vi "_AppData.Test Class.vi"() -> ()   [LabVIEW 2024, in "EQMF.lvlib" / "Config Utils.lvlib"]
uses:
  Config Utils.lvlib
  Class.AppData.lvclass
  <vilib>/Utility/sysdir.llb/System Directory Type.ctl
panel:
  out "App Data Folder":path
  out "Replaced 3":bool
  out "Replaced 2":bool
  out "Replaced 1":bool
  out "Found 3":bool
  out "Found 2":bool
  out "Found 1":bool
  out "error out":errorcluster
  in  "Store and Exit":bool
  in  "Init":bool
  in  "Get 3":bool
  in  "Get 2":bool
  in  "Get 1":bool
  in  "Save 3":bool
  in  "Save 2":bool
  in  "Save 1":bool
  in  "Data 3":bool
  in  "Data 2":T1
  in  "Data 1":dbl
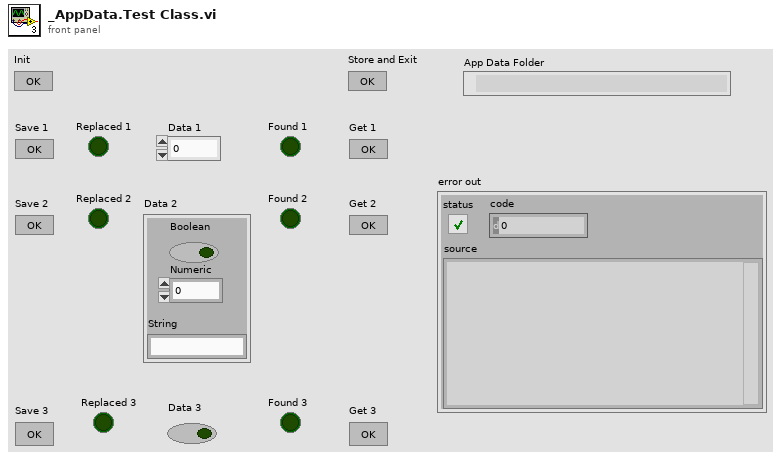
[diagram p1: front panel]
types:
  T1 = cluster{"Boolean":bool, "Numeric":dbl, "String":string}
  T2 = typedef "System Directory Type.ctl" = i32
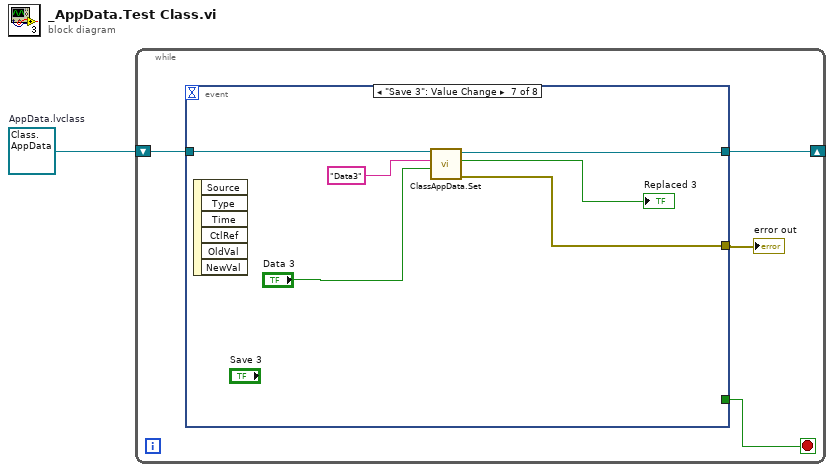
[diagram p0: block diagram]
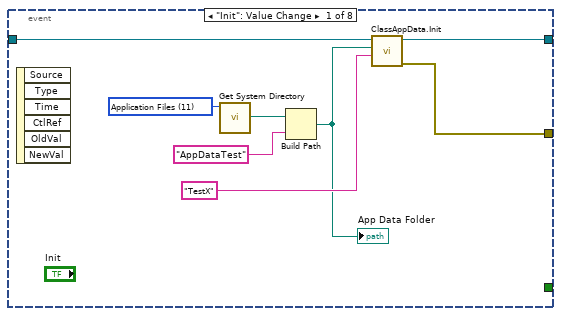
[diagram p2: hidden frame]
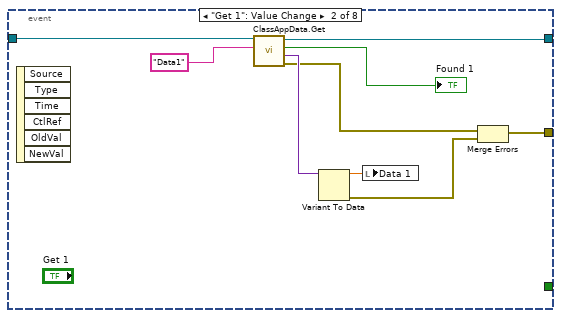
[diagram p3: hidden frame]
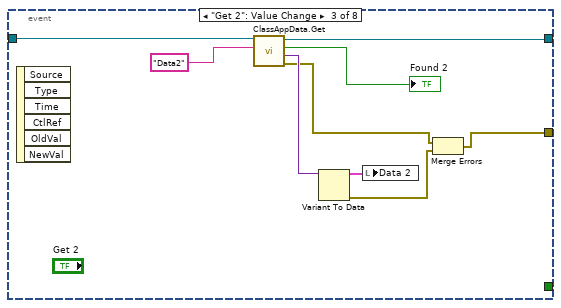
[diagram p4: hidden frame]
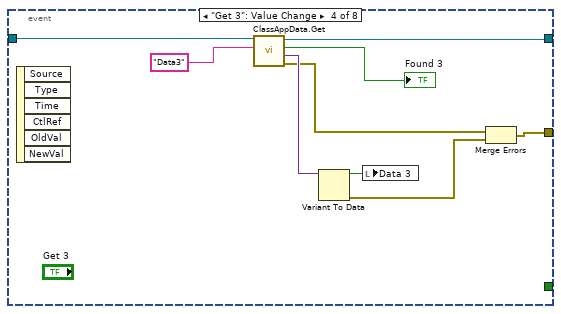
[diagram p5: hidden frame]
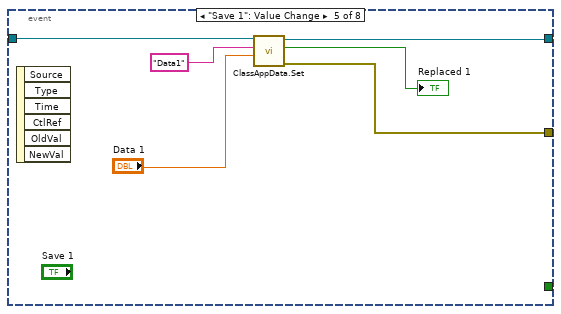
[diagram p6: hidden frame]
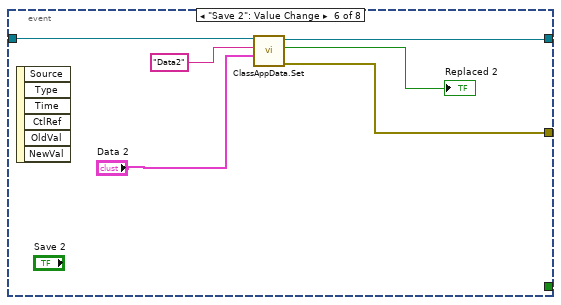
[diagram p7: hidden frame]
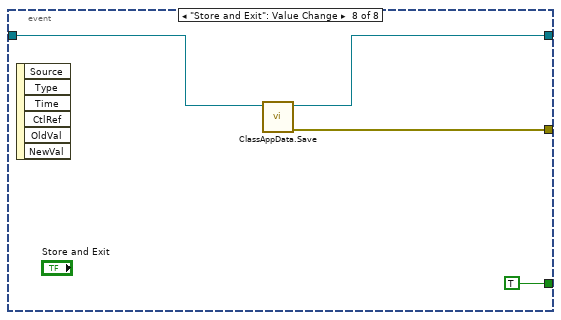
[diagram p8: hidden frame]
diagram:
  w1 = refnum<class "Class.AppData.lvclass"> refnum  # AppData.lvclass
  n1 = while {
    shift-right: [w4] -> _
    shift-left: w1 -> [w5]
    stop <- w3 stop-if-true
    n2 = event shown="[6] \"Save 3\": Value Change" {
      selector: _ -> [_ _ _ _ _ _ _ _]
      dyn-events: _ -> [_ _ _ _ _ _ _ _]
      timeout: _ -> [_ _ _ _ _ _ _ _]
      tunnel: w5 -> [w13 w22 w31 w40 w46 w52 w58 w61]
      tunnel: [w12 w21 w30 w39 w45 w51 w57 w60] -> w4
      tunnel: [_ _ _ _ _ _ _ TRUE] -> w3
      tunnel: [w6 w16 w23 w34 w44 w50 w56 w59] -> w2
      event "Init": Value Change {
        w11 = T2 11 items=["User Home"=0, "User Desktop"=1, "User Documents"=2, "User Application Data"=3, "User Preferences"=4, "User Temporary"=5, "Public Documents"=6, "Public Application Data"=7, "Public Preferences"=8, "Public Cache"=13, "System Core Libraries"=9, "System Installed Libraries"=10, "Application Files"=11, "Boot Volume Root"=12] ("system directory type")
        n3 = event-data() -> ()  [unwired: 1 in, 6 out]
        n4 = call <vilib>:"Get System Directory.vi"("system directory type"=w11) -> ("system directory"=w10:path)  [unwired: 10 in]
        n5 = Build Path(base path=w10, name or relative path="AppDataTest") -> (appended path=w7:path)
        "App Data Folder" <- w7
        n6 = call "ClassAppData.Init.vi"("Module Name"="TestX", "App Data Dir"=w7, "Class - App Data in"=w13) -> ("error out"=w6:errorcluster, "Class - App Data out"=w12:refnum<class "Class.AppData.lvclass">)  [unwired: 6 in, 1 out]
      }
      event "Get 1": Value Change {
        n7 = event-data() -> ()  [unwired: 1 in, 6 out]
        n8 = call "ClassAppData.Get.vi"("Section"="Data1" ("Data Name"), "Class - App Data in"=w22) -> ("error out"=w15:errorcluster, "Data Out"=w20:variant, "Found"=→"Found 1":bool, "Class - App Data out"=w21:refnum<class "Class.AppData.lvclass">)  [unwired: 5 in, 1 out]
        n9 = Variant To Data(Variant=w20) -> (data=w19:dbl, error out=w14:errorcluster)  [unwired: 2 in]
        n10 = local write "Data 1"(w19) -> ()
        n11 = Merge Errors(w15, w14) -> (w16:errorcluster)
      }
      event "Get 2": Value Change {
        n12 = event-data() -> ()  [unwired: 1 in, 6 out]
        n13 = call "ClassAppData.Get.vi"("Section"="Data2" ("Data Name"), "Class - App Data in"=w31) -> ("error out"=w25:errorcluster, "Data Out"=w29:variant, "Found"=→"Found 2":bool, "Class - App Data out"=w30:refnum<class "Class.AppData.lvclass">)  [unwired: 5 in, 1 out]
        n14 = Variant To Data(Variant=w29) -> (data=w28:T1, error out=w24:errorcluster)  [unwired: 2 in]
        n15 = local write "Data 2"(w28) -> ()
        n16 = Merge Errors(w25, w24) -> (w23:errorcluster)
      }
      event "Get 3": Value Change {
        n17 = event-data() -> ()  [unwired: 1 in, 6 out]
        n18 = call "ClassAppData.Get.vi"("Section"="Data3" ("Data Name"), "Class - App Data in"=w40) -> ("error out"=w33:errorcluster, "Data Out"=w38:variant, "Found"=→"Found 3":bool, "Class - App Data out"=w39:refnum<class "Class.AppData.lvclass">)  [unwired: 5 in, 1 out]
        n19 = Variant To Data(Variant=w38) -> (data=w37:bool, error out=w32:errorcluster)  [unwired: 2 in]
        n20 = local write "Data 3"(w37) -> ()
        n21 = Merge Errors(w33, w32) -> (w34:errorcluster)
      }
      event "Save 1": Value Change {
        n22 = event-data() -> ()  [unwired: 1 in, 6 out]
        n23 = call "ClassAppData.Set.vi"("Value"="Data 1", "Name"="Data1" ("Data Name"), "Class - App Data in"=w46) -> ("error out"=w44:errorcluster, "Replaced"=→"Replaced 1":bool, "Class - App Data out"=w45:refnum<class "Class.AppData.lvclass">)  [unwired: 6 in]
      }
      event "Save 2": Value Change {
        n24 = event-data() -> ()  [unwired: 1 in, 6 out]
        n25 = call "ClassAppData.Set.vi"("Value"="Data 2", "Name"="Data2" ("Data Name"), "Class - App Data in"=w52) -> ("error out"=w50:errorcluster, "Replaced"=→"Replaced 2":bool, "Class - App Data out"=w51:refnum<class "Class.AppData.lvclass">)  [unwired: 6 in]
      }
      event "Save 3": Value Change {
        n26 = event-data() -> ()  [unwired: 1 in, 6 out]
        n27 = call "ClassAppData.Set.vi"("Value"="Data 3", "Name"="Data3" ("Data Name"), "Class - App Data in"=w58) -> ("error out"=w56:errorcluster, "Replaced"=→"Replaced 3":bool, "Class - App Data out"=w57:refnum<class "Class.AppData.lvclass">)  [unwired: 6 in]
      }
      event "Store and Exit": Value Change {
        n28 = event-data() -> ()  [unwired: 1 in, 6 out]
        n29 = call "ClassAppData.Save.vi"("Class - App Data in"=w61) -> ("error out"=w59:errorcluster, "Class - App Data out"=w60:refnum<class "Class.AppData.lvclass">)  [unwired: 9 in]
      }
    }
    "error out" <- w2
  }
